vi "get_max_iter.vi"(8 "error in":errorcluster, 10 "date_str":string="20180206", 11 "base":path) -> (0 "error out":errorcluster, 1 "num_folders":i32, 2 "max ID":i32, 3 "IDS":i32[](array[numeric]), 4 "path":path, 5 "folder names":string[](array[string]))   [LabVIEW 2017, in "tools.lvlib"]
uses:
  tools.lvlib
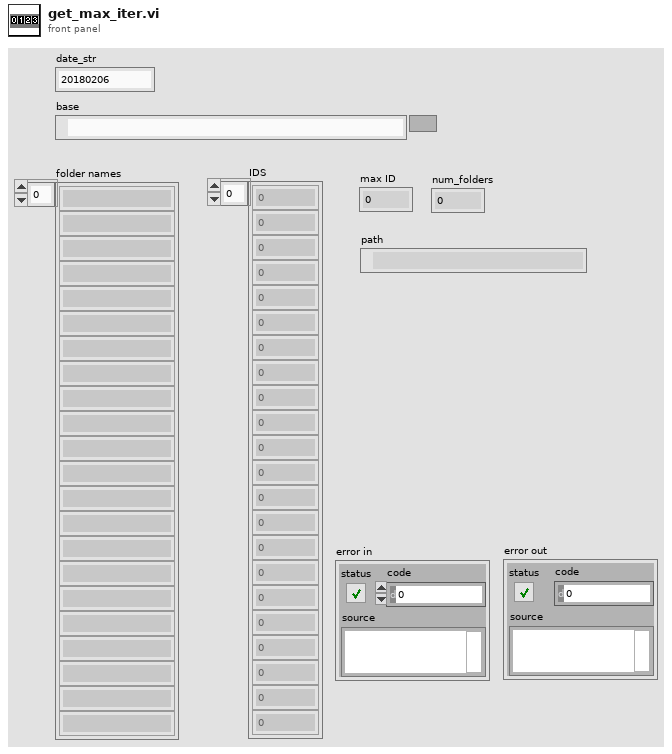
[diagram p1: front panel]
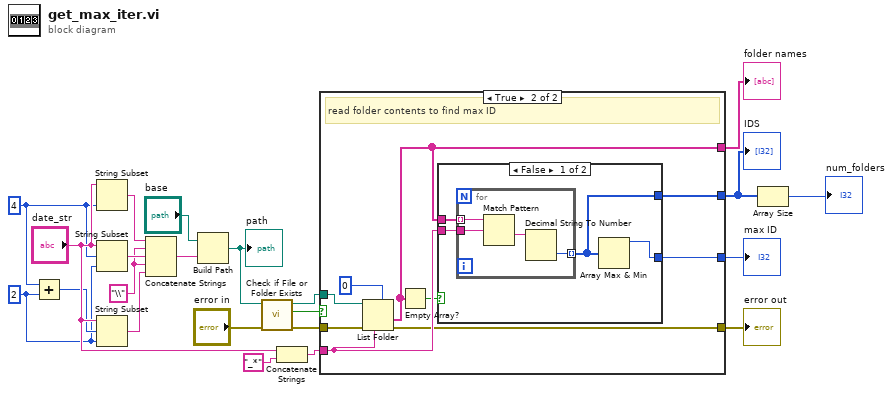
[diagram p0: block diagram]
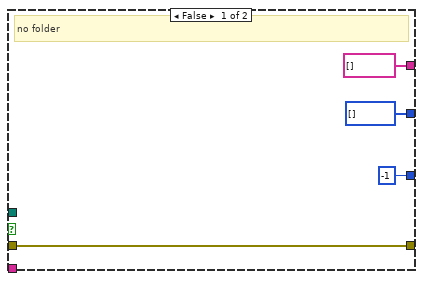
[diagram p2: hidden frame]
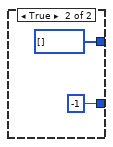
[diagram p3: hidden frame]
diagram:
  w12 = "\\" ("string")
  w16 = 2 ("length (rest)")
  w18 = 4 ("length (rest)")
  n1 = Add(x=w18, y=w16) -> (x+y=w17:i32)
  n2 = String Subset(string="date_str", length (rest)=w18) -> (substring=w15:string)  [unwired: 1 in]
  n3 = String Subset(string="date_str", offset (0)=w18, length (rest)=w16) -> (substring=w14:string)
  n4 = String Subset(string="date_str", offset (0)=w17, length (rest)=w16) -> (substring=w13:string)
  n5 = Concatenate Strings(w15, w12, w14, w12, w13) -> (w11:string)
  n6 = Build Path(base path="base", name or relative path=w11) -> (appended path=w10:path)
  "path" <- w10
  n7 = call <vilib>:"Check if File or Folder Exists.vi"("error in (no error)"="error in", "path"=w10) -> ("error out"=w6:errorcluster, "file or folder exists?"=w8:bool, "dup path"=w7:path)  [unwired: 7 in]
  n8 = Concatenate Strings("date_str", "_*" ("string")) -> (w21:string)
  n9 = case shown="True" w8 {
    tunnel: w21 -> [_ w34]
    tunnel: w7 -> [_ w33]
    tunnel: w6 -> [w26 w32]
    tunnel: [w26 w31] -> w5
    tunnel: [-1 w28] -> w4
    tunnel: [i32[] [] w27] -> w2
    tunnel: [string[] [] ("folder names") w30] -> w3
    frame False {
      # "no folder"
    }
    frame True {
      # "read folder contents to find max ID"
      n10 = List Folder(datalog type=0, path=w33, pattern=w34, error in=w32) -> (folder names=w30:string[], error out=w31:errorcluster)  [unwired: 2 out]
      n11 = Empty Array?(array=w30) -> (empty?=w29:bool)
      n12 = case shown="False" w29 {
        tunnel: w34 -> [w39 _]
        tunnel: [w37 -1] -> w28
        tunnel: w30 -> [w38 _]
        tunnel: [w36 i32[] []] -> w27
        frame False {
          n13 = for {
            tunnel: w38 -> [w43] mode=indexing
            tunnel: w39 -> [w42]
            tunnel: [w40] -> w36 mode=indexing
            n14 = Match Pattern(string=w43, regular expression=w42) -> (after substring=w41:string)  [unwired: 1 in, 3 out]
            n15 = Decimal String To Number(string=w41) -> (number=w40:i32)  [unwired: 2 in, 1 out]
          }
          n16 = Array Max & Min(array=w36) -> (max value=w37:i32)  [unwired: 3 out]
        }
        frame True {
        }
      }
    }
  }
  "error out" <- w5
  "max ID" <- w4
  "IDS" <- w2
  "folder names" <- w3
  n17 = Array Size(array=w2) -> (size(s)=→"num_folders":i32)
